vi "PM5000_v3.vi"() -> ()   [LabVIEW 2018]
uses:
  <vilib>/addons/database/Connection.llb/DB Tools Open Connec (Path).vi
  Global/Demo.vi
  Global/estadoGeneradores.vi
  <vilib>/addons/database/NI_Database_API.lvlib
panel:
  out "codeG6":i32
  out "codeG5":i32
  out "codeG4":i32
  out "codeG3":i32
  out "codeG2":i32
  out "codeG1":i32
  out "G6":string
  out "G5":string
  out "G4":string
  out "G3":string
  out "G2":string
  out "G1":string
  out "ID G6":i32
  out "ID G5":i32
  out "ID G4":i32
  out "ID G3":i32
  out "ID G2":i32
  out "ID_G1":i32
  out "error out":errorcluster
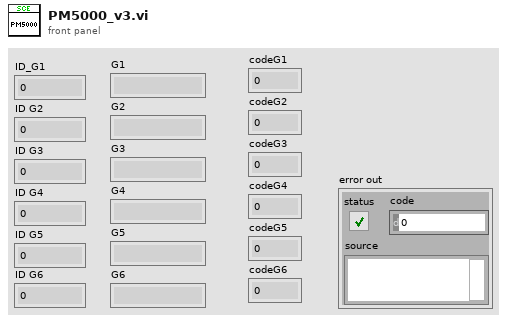
[diagram p1: front panel]
types:
  T1 = typedef "NI_Database_API.lvlib/Conn ObjectReference.ctl" = refnum<k1>
  T2 = typedef "Equipos_Medicion_cluster.ctl" = cluster{"ID_EQUIPO":i32, "IP_EQUIPO":string, "NOMBRE_EQUIPO":string, "ESTADO_EQUIPO":string, "DESCRIPCION":string, "ID_MEDICION":i32, "ESTADO_MEDICION":string, "TIEMPO_MEDICION":string}
  T3 = typedef "Cluster_Data.ctl" = cluster{"Equipo_Medicion":T2, "VIF_cluster":T4, "Power_cluster":T5, "THD_cluster":T6, "Polar_cluster":T7}
  T4 = typedef "VIF_cluster.ctl" = cluster{"VL_VL":cluster{"V1_V2":sgl, "V2_V3":sgl, "V3_V1":sgl, "Avg_VL_VL":sgl}, "IL_IL":cluster{"I1":sgl, "I2":sgl, "I3":sgl, "Avg_Amps":sgl}, "Frecuency":sgl, "Avg_Frecuency":sgl}
  T5 = typedef "Power_cluster.ctl" = cluster{"Real Power (kW)":cluster{"L1_kW":sgl, "L2_kW":sgl, "L3_kW":sgl, "Total_kW":sgl}, "Reactive Power (kVAR)":cluster{"L1_kVAR":sgl, "L2_kVAR":sgl, "L3_kVAR":sgl, "Total_kVAR":sgl}, "Aparent Power (kVA)":cluster{"L1_kVA":sgl, "L2_kVA":sgl, "L3_kVA":sgl, "Total_kVA":sgl}, "Power Factor (%)":cluster{"L1_PF":sgl, "L2_PF":sgl, "L3_PF":sgl, "Total_PF":sgl}}
  T6 = typedef "THD_cluster.ctl" = cluster{"V_THD":cluster{"V1_V2_THD":sgl, "V2_V3_THD":sgl, "V3_V1_THD":sgl, "Avg_V_V_THD":sgl}, "I_THD":cluster{"I1_THD":sgl, "I2_THD":sgl, "I3_THD":sgl, "I4_THD":sgl, "Avg_I_THD":sgl}}
  T7 = typedef "Polar_cluster.ctl" = cluster{"V_polar":cluster{"V1_ang":sgl, "V1_mag":sgl, "V2_ang":sgl, "V2_mag":sgl, "V3_ang":sgl, "V3_mag":sgl}, "I_polar":cluster{"I1_ang":sgl, "I1_mag":sgl, "I2_ang":sgl, "I2_mag":sgl, "I3_ang":sgl, "I3_mag":sgl}}
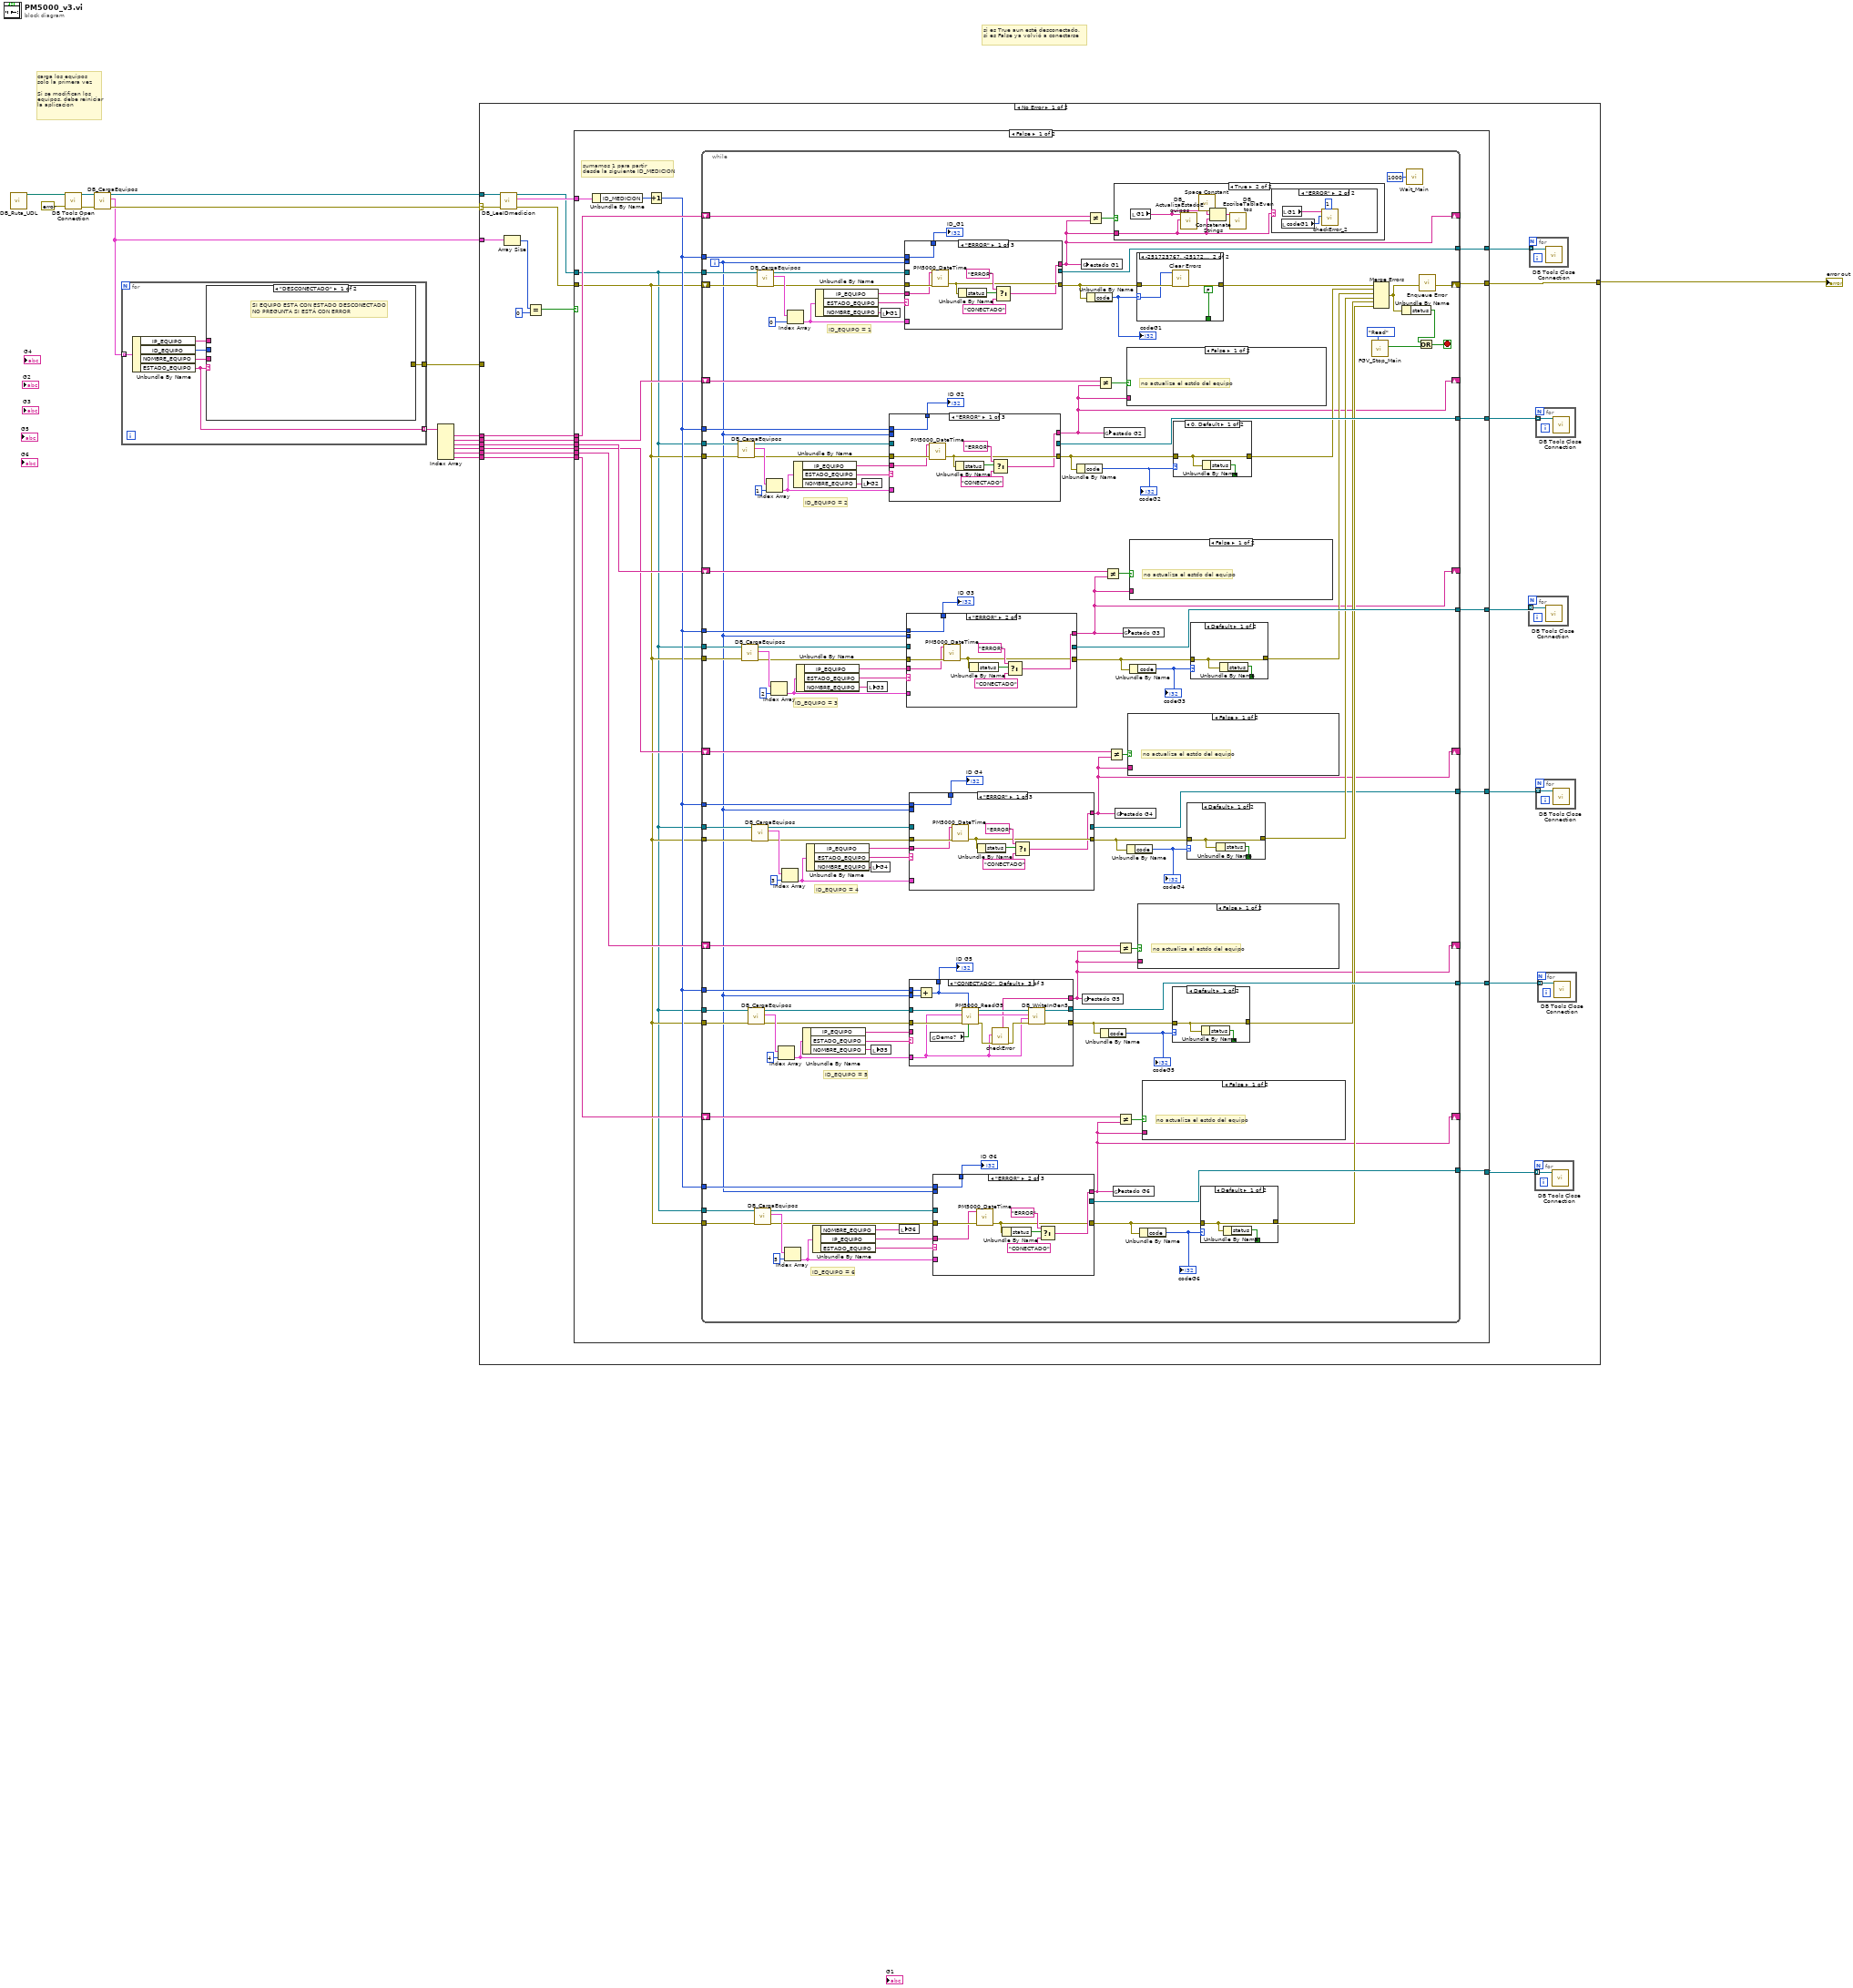
[diagram p0: block diagram]
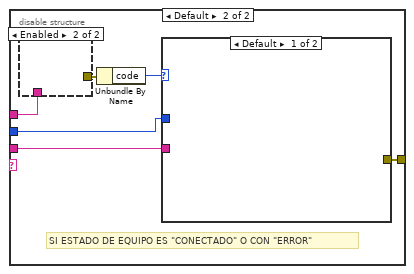
[diagram p2: hidden frame]
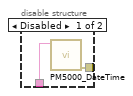
[diagram p3: hidden frame]
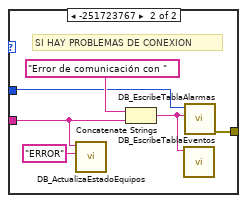
[diagram p4: hidden frame]
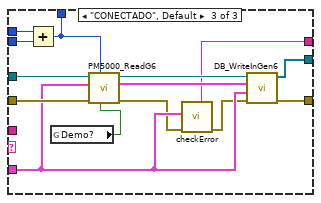
[diagram p6: hidden frame]
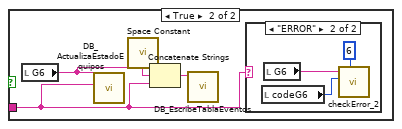
[diagram p7: hidden frame]
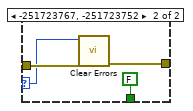
[diagram p9: hidden frame]
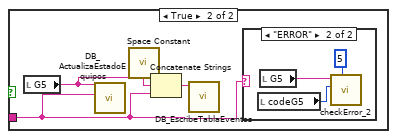
[diagram p10: hidden frame]
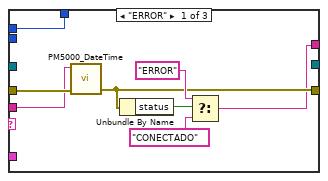
[diagram p12: hidden frame]
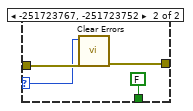
[diagram p14: hidden frame]
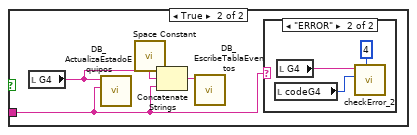
[diagram p15: hidden frame]
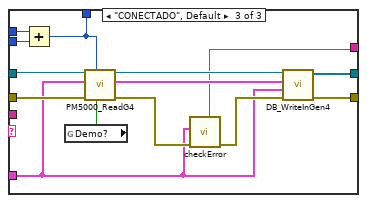
[diagram p18: hidden frame]
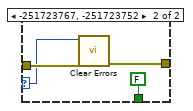
[diagram p19: hidden frame]
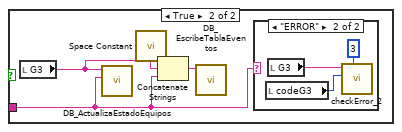
[diagram p20: hidden frame]
diagram:
  # "si es True aun esté desconectado.\nsi es False ya volvió a conectarse"
  # "carga los equipos\nsolo la primera vez\n\nSi se modifican los\nequipos, debe reiniciar\nla aplicacion"
  n1 = call "DB_Ruta_UDL.vi"() -> ("UDL ruta"=w14:path)  [unwired: 11 in]
  n2 = call-poly <vilib>:"DB Tools Open Connection.vi"("error in (no error)"=errorcluster {"status"=FALSE, "code"=0, "source"=""}, "connection information"=w14) -> ("error out"=w12:errorcluster, "connection reference"=w13:T1)  [unwired: 6 in]
  n3 = call "DB_CargaEquipos.vi"("error in (no error)"=w12, "db in"=w13) -> ("error out"=w10:errorcluster, "Equipos_out"=w9:T2[], "db out"=w11:T1)  [unwired: 2 in, 5 out]
  n4 = for {
    tunnel: w9 -> [w22] mode=indexing
    tunnel: [w20] -> w8
    tunnel: [w17] -> w7 mode=indexing
    n5 = Unbundle By Name(w22) -> ("IP_EQUIPO"=w19:string, "ID_EQUIPO"=w21:i32, "NOMBRE_EQUIPO"=w18:string, "ESTADO_EQUIPO"=w17:string)
    n6 = case shown="\"DESCONECTADO\"" w17 {
      tunnel: w21 -> [_ w26]
      tunnel: [_ w25] -> w20
      tunnel: w19 -> [_ w24]
      tunnel: w18 -> [_ w23]
      frame "DESCONECTADO" {
        # "SI EQUIPO ESTA CON ESTADO DESCONECTADO\nNO PREGUNTA SI ESTÁ CON ERROR"
      }
      frame Default {
        # "SI ESTADO DE EQUIPO ES \"CONECTADO\" O CON \"ERROR\""
        n7 = disable-structure shown="Enabled" {
          disable-tunnel: [w30 _] -> w28
          disable-tunnel: w24 -> [w29 _]
          frame Disabled {
            n8 = call "PM5000_DateTime.vi"("Network Path"=w29) -> ("error out"=w30:errorcluster)  [unwired: 7 in, 3 out]
          }
          frame Enabled {
          }
        }
        n9 = Unbundle By Name(w28) -> ("code"=w27:i32)
        n10 = case shown="Default" w27 {
          tunnel: w23 -> [_ w31]
          tunnel: w26 -> [_ w34]
          tunnel: [_ w33] -> w25
          frame Default {
          }
          frame -251723767 {
            # "SI HAY PROBLEMAS DE CONEXION"
            n11 = call "DB_ActualizaEstadoEquipos.vi"("ESTADO_EQUIPO"="ERROR", "NOMBRE_EQUIPO"=w31) -> ()  [unwired: 9 in, 1 out]
            n12 = Concatenate Strings("Error de comunicación con " ("string"), w31) -> (w35:string)
            n13 = call "DB_EscribeTablaEventos.vi"("DESCRIPCION"=w35) -> ()  [unwired: 10 in, 1 out]
            n14 = call "DB_EscribeTablaAlarmas.vi"("MOTIVO"=w35, "ID_EQUIPO"=w34) -> ("error out"=w33:errorcluster)  [unwired: 9 in]
          }
        }
      }
    }
  }
  n15 = Index Array(array=w7) -> (element #1=w5:string, element #2=w4:string, element #3=w3:string, element #4=w2:string, element #5=w1:string, element #6=w6:string)  [unwired: 6 in]
  n16 = case shown="No Error" w10 {
    selector: w10 -> [w44 w428]
    tunnel: [w58 w427] -> w15
    tunnel: w9 -> [w55 _]
    tunnel: w11 -> [w51 _]
    tunnel: w8 -> [_ _]
    tunnel: w6 -> [w43 _]
    tunnel: w5 -> [w41 _]
    tunnel: w4 -> [w40 _]
    tunnel: w3 -> [w39 _]
    tunnel: w2 -> [w38 _]
    tunnel: w1 -> [w37 _]
    frame No Error {
      n17 = call "DB_LeeIDmedicion.vi"("error in (no error)"=w44, "db in"=w51) -> ("error out"=w46:errorcluster, "Equipo_Medicion out"=w50:T2, "db out"=w45:T1)  [unwired: 7 in]
      n18 = Array Size(array=w55) -> (size(s)=w56:i32)
      n19 = Equal?(x=w56, y=0) -> (x = y?=w54:bool)
      n20 = case shown="False" w54 {
        tunnel: [w75 w426] -> w58
        tunnel: w46 -> [w66 w426]
        tunnel: w45 -> [w65 _]
        tunnel: [w82 _] -> w53
        tunnel: [w81 _] -> w52
        tunnel: w50 -> [w80 _]
        tunnel: [w78 _] -> w49
        tunnel: [w77 _] -> w48
        tunnel: [w76 _] -> w47
        tunnel: w43 -> [w74 _]
        tunnel: [w73 _] -> w42
        tunnel: w41 -> [w72 _]
        tunnel: w40 -> [w71 _]
        tunnel: w39 -> [w70 _]
        tunnel: w38 -> [w69 _]
        tunnel: w37 -> [w68 _]
        frame False {
          # "sumamos 1 para partir\ndesde la siguiente ID_MEDICION"
          n21 = Unbundle By Name(w80) -> ("ID_MEDICION"=w79:i32)
          n22 = Increment(x=w79) -> (x+1=w67:i32)
          n23 = while {
            tunnel: [w204] -> w82
            tunnel: [w203] -> w81
            tunnel: [w202] -> w78
            tunnel: [w201] -> w77
            tunnel: [w200] -> w76
            tunnel: w65 -> [w199]
            tunnel: [w189] -> w73
            tunnel: w67 -> [w112]
            shift-right: [w197] -> w75
            shift-left: w66 -> [w198]
            tunnel: w67 -> [w110]
            tunnel: w67 -> [w106]
            tunnel: w67 -> [w105]
            tunnel: w67 -> [w104]
            tunnel: w67 -> [w103]
            tunnel: w66 -> [w102]
            tunnel: w66 -> [w101]
            tunnel: w66 -> [w100]
            tunnel: w66 -> [w99]
            tunnel: w66 -> [w98]
            tunnel: w65 -> [w97]
            tunnel: w65 -> [w96]
            tunnel: w65 -> [w95]
            tunnel: w65 -> [w94]
            tunnel: w65 -> [w93]
            shift-right: [w91] -> _
            shift-left: w72 -> [w188]
            shift-right: [w90] -> _
            shift-left: w71 -> [w187]
            shift-right: [w89] -> _
            shift-left: w70 -> [w186]
            shift-right: [w88] -> _
            shift-left: w69 -> [w185]
            shift-right: [w87] -> _
            shift-left: w68 -> [w184]
            shift-right: [w86] -> _
            shift-left: w74 -> [w190]
            i -> [w92]
            stop <- w107 stop-if-true
            # "ID_EQUIPO = 6"
            # "ID_EQUIPO = 5"
            # "ID_EQUIPO = 4"
            # "ID_EQUIPO = 3"
            # "ID_EQUIPO = 2"
            # "ID_EQUIPO = 1"
            n24 = call "DB_CargaEquipos.vi"("error in (no error)"=w102, "db in"=w97) -> ("error out"=w168:errorcluster, "Equipos_out"=w171:T2[], "db out"=w170:T1)  [unwired: 2 in, 5 out]
            n25 = call "DB_CargaEquipos.vi"("error in (no error)"=w101, "db in"=w96) -> ("error out"=w156:errorcluster, "Equipos_out"=w159:T2[], "db out"=w158:T1)  [unwired: 2 in, 5 out]
            n26 = call "DB_CargaEquipos.vi"("error in (no error)"=w99, "db in"=w94) -> ("error out"=w134:errorcluster, "Equipos_out"=w137:T2[], "db out"=w136:T1)  [unwired: 2 in, 5 out]
            n27 = call "DB_CargaEquipos.vi"("error in (no error)"=w100, "db in"=w95) -> ("error out"=w145:errorcluster, "Equipos_out"=w148:T2[], "db out"=w147:T1)  [unwired: 2 in, 5 out]
            n28 = call "DB_CargaEquipos.vi"("error in (no error)"=w98, "db in"=w93) -> ("error out"=w120:errorcluster, "Equipos_out"=w123:T2[], "db out"=w122:T1)  [unwired: 2 in, 5 out]
            n29 = call "DB_CargaEquipos.vi"("error in (no error)"=w198, "db in"=w199) -> ("error out"=w179:errorcluster, "Equipos_out"=w182:T2[], "db out"=w181:T1)  [unwired: 2 in, 5 out]
            n30 = Index Array(array=w171, index=1) -> (element=w167:T2)
            n31 = Index Array(array=w159, index=2) -> (element=w155:T2)
            n32 = Index Array(array=w137, index=4) -> (element=w133:T2)
            n33 = Index Array(array=w148, index=3) -> (element=w144:T2)
            n34 = Index Array(array=w123, index=5) -> (element=w119:T2)
            n35 = Index Array(array=w182, index=0) -> (element=w178:T2)
            n36 = Unbundle By Name(w167) -> ("IP_EQUIPO"=w164:string, "ESTADO_EQUIPO"=w166:string, "NOMBRE_EQUIPO"=w161:string)
            n37 = Unbundle By Name(w155) -> ("IP_EQUIPO"=w152:string, "ESTADO_EQUIPO"=w154:string, "NOMBRE_EQUIPO"=w150:string)
            n38 = Unbundle By Name(w133) -> ("IP_EQUIPO"=w130:string, "ESTADO_EQUIPO"=w132:string, "NOMBRE_EQUIPO"=w126:string)
            n39 = Unbundle By Name(w144) -> ("IP_EQUIPO"=w142:string, "ESTADO_EQUIPO"=w143:string, "NOMBRE_EQUIPO"=w140:string)
            n40 = Unbundle By Name(w119) -> ("NOMBRE_EQUIPO"=w116:string, "IP_EQUIPO"=w117:string, "ESTADO_EQUIPO"=w118:string)
            n41 = Unbundle By Name(w178) -> ("IP_EQUIPO"=w176:string, "ESTADO_EQUIPO"=w177:string, "NOMBRE_EQUIPO"=w175:string)
            n42 = local write "G2"(w161) -> ()
            n43 = local write "G3"(w150) -> ()
            n44 = local write "G4"(w140) -> ()
            n45 = local write "G5"(w126) -> ()
            n46 = local write "G1"(w175) -> ()
            n47 = case shown="\"ERROR\"" w166 {
              selector: w166 -> [_ w369 _]
              tunnel: [_ _ w382] -> w203
              tunnel: w170 -> [_ _ w380]
              tunnel: w167 -> [_ _ w373]
              tunnel: [w367 w368 w376] -> w165
              tunnel: w168 -> [w363 _ w379]
              tunnel: [w361 _ w378] -> w172
              tunnel: [w360 w369 w372] -> w90
              tunnel: w112 -> [w367 w368 w377]
              tunnel: w164 -> [w362 _ _]
              tunnel: w92 -> [_ _ w371]
              frame "ERROR" {
                n48 = call "PM5000_DateTime.vi"("error in"=w363, "Network Path"=w362) -> ("error out"=w361:errorcluster)  [unwired: 6 in, 3 out]
                n49 = Unbundle By Name(w361) -> ("status"=w366:bool)
                n50 = Select(t="ERROR", s=w366, f="CONECTADO") -> (s? t:f=w360:string)
              }
              frame "DESCONECTADO" {
              }
              frame "CONECTADO", Default {
                n51 = Add(x=w377, y=w371) -> (x+y=w376:i32)
                n52 = global read "Demo.vi" "Demo?"() -> (w370:bool)
                n53 = call "PM5000_ReadG2.vi"("DEMO"=w370, "ID_MEDICION"=w376, "error in (no error)"=w379, "Equipo_Medicion"=w373) -> ("error out"=w375:errorcluster, "PM_out"=w381:T3)  [unwired: 6 in]
                n54 = call "checkError.vi"("error in (no error)"=w375, "Equipo_Medicion in"=w373) -> ("error out"=w374:errorcluster, "ESTADO_EQUIPO"=w372:string)  [unwired: 8 in]
                n55 = call "DB_WriteInGen2.vi"("error in (no error)"=w374, "Equipo_Medicion"=w373, "PM_out"=w381, "DB in"=w380) -> ("error out"=w378:errorcluster, "closeDB"=w382:T1[])  [unwired: 6 in]
              }
            }
            "ID G2" <- w165
            n56 = local write "G6"(w116) -> ()
            n57 = case shown="\"ERROR\"" w177 {
              selector: w177 -> [_ w406 _]
              tunnel: [_ _ w419] -> w204
              tunnel: w181 -> [_ _ w418]
              tunnel: w179 -> [w400 w405 w416]
              tunnel: [w399 w405 w415] -> w183
              tunnel: w178 -> [_ _ w408]
              tunnel: w176 -> [w396 _ _]
              tunnel: [w398 w406 w412] -> w91
              tunnel: [w397 w404 w411] -> w113
              tunnel: w110 -> [w397 w404 w410]
              tunnel: w92 -> [_ _ w409]
              frame "ERROR" {
                n58 = call "PM5000_DateTime.vi"("error in"=w400, "Network Path"=w396) -> ("error out"=w399:errorcluster)  [unwired: 6 in, 3 out]
                n59 = Unbundle By Name(w399) -> ("status"=w403:bool)
                n60 = Select(t="ERROR", s=w403, f="CONECTADO") -> (s? t:f=w398:string)
              }
              frame "DESCONECTADO" {
              }
              frame "CONECTADO", Default {
                n61 = Add(x=w410, y=w409) -> (x+y=w411:i32)
                n62 = global read "Demo.vi" "Demo?"() -> (w407:bool)
                n63 = call "PM5000_ReadG1.vi"("DEMO"=w407, "ID_MEDICION"=w411, "error in (no error)"=w416, "Equipo_Medicion"=w408) -> ("error out"=w414:errorcluster, "PM_out"=w417:T3)  [unwired: 6 in]
                n64 = call "checkError.vi"("error in (no error)"=w414, "Equipo_Medicion in"=w408) -> ("error out"=w413:errorcluster, "ESTADO_EQUIPO"=w412:string)  [unwired: 8 in]
                n65 = call "DB_WriteInGen1.vi"("error in (no error)"=w413, "Equipo_Medicion"=w408, "PM_out"=w417, "DB in"=w418) -> ("error out"=w415:errorcluster, "closeDB"=w419:T1[])  [unwired: 6 in]
              }
            }
            "ID_G1" <- w113
            n66 = case shown="\"ERROR\"" w154 {
              selector: w154 -> [_ _ w346]
              tunnel: [w335 _ _] -> w202
              tunnel: w158 -> [w333 _ _]
              tunnel: w155 -> [w326 _ _]
              tunnel: w156 -> [w332 w340 w345]
              tunnel: [w331 w337 w345] -> w160
              tunnel: [w327 w338 w346] -> w89
              tunnel: [w330 w336 w344] -> w153
              tunnel: w152 -> [_ w339 _]
              tunnel: w106 -> [w325 w336 w344]
              tunnel: w92 -> [w324 _ _]
              frame "CONECTADO", Default {
                n67 = Add(x=w325, y=w324) -> (x+y=w330:i32)
                n68 = global read "Demo.vi" "Demo?"() -> (w323:bool)
                n69 = call "PM5000_ReadG3.vi"("DEMO"=w323, "ID_MEDICION"=w330, "error in (no error)"=w332, "Equipo_Medicion"=w326) -> ("error out"=w329:errorcluster, "PM_out"=w334:T3)  [unwired: 6 in]
                n70 = call "checkError.vi"("error in (no error)"=w329, "Equipo_Medicion in"=w326) -> ("error out"=w328:errorcluster, "ESTADO_EQUIPO"=w327:string)  [unwired: 8 in]
                n71 = call "DB_WriteInGen3.vi"("error in (no error)"=w328, "Equipo_Medicion"=w326, "PM_out"=w334, "DB in"=w333) -> ("error out"=w331:errorcluster, "closeDB"=w335:T1[])  [unwired: 6 in]
              }
              frame "ERROR" {
                n72 = call "PM5000_DateTime.vi"("error in"=w340, "Network Path"=w339) -> ("error out"=w337:errorcluster)  [unwired: 6 in, 3 out]
                n73 = Unbundle By Name(w337) -> ("status"=w343:bool)
                n74 = Select(t="ERROR", s=w343, f="CONECTADO") -> (s? t:f=w338:string)
              }
              frame "DESCONECTADO" {
              }
            }
            "ID G3" <- w153
            n75 = case shown="\"CONECTADO\", Default" w132 {
              selector: w132 -> [_ w258 _]
              tunnel: [_ _ w272] -> w201
              tunnel: w136 -> [_ _ w270]
              tunnel: w133 -> [_ _ w264]
              tunnel: w134 -> [w253 w259 w269]
              tunnel: [w251 w259 w268] -> w129
              tunnel: [w250 w258 w263] -> w87
              tunnel: [w249 w257 w267] -> w131
              tunnel: w130 -> [w252 _ _]
              tunnel: w104 -> [w249 w257 w262]
              tunnel: w92 -> [_ _ w261]
              frame "ERROR" {
                n76 = call "PM5000_DateTime.vi"("error in"=w253, "Network Path"=w252) -> ("error out"=w251:errorcluster)  [unwired: 6 in, 3 out]
                n77 = Unbundle By Name(w251) -> ("status"=w256:bool)
                n78 = Select(t="ERROR", s=w256, f="CONECTADO") -> (s? t:f=w250:string)
              }
              frame "DESCONECTADO" {
              }
              frame "CONECTADO", Default {
                n79 = Add(x=w262, y=w261) -> (x+y=w267:i32)
                n80 = global read "Demo.vi" "Demo?"() -> (w260:bool)
                n81 = call "PM5000_ReadG5.vi"("DEMO"=w260, "ID_MEDICION"=w267, "error in (no error)"=w269, "Equipo_Medicion"=w264) -> ("error out"=w266:errorcluster, "PM_out"=w271:T3)  [unwired: 6 in]
                n82 = call "checkError.vi"("error in (no error)"=w266, "Equipo_Medicion in"=w264) -> ("error out"=w265:errorcluster, "ESTADO_EQUIPO"=w263:string)  [unwired: 8 in]
                n83 = call "DB_WriteInGen5.vi"("error in (no error)"=w265, "Equipo_Medicion"=w264, "PM_out"=w271, "DB in"=w270) -> ("error out"=w268:errorcluster, "closeDB"=w272:T1[])  [unwired: 6 in]
              }
            }
            "ID G5" <- w131
            n84 = case shown="\"ERROR\"" w143 {
              selector: w143 -> [_ w296 _]
              tunnel: [_ _ w309] -> w189
              tunnel: w147 -> [_ _ w307]
              tunnel: w144 -> [_ _ w302]
              tunnel: w145 -> [w290 w295 w306]
              tunnel: [w289 w295 w305] -> w139
              tunnel: [w288 w296 w301] -> w88
              tunnel: w142 -> [w287 _ _]
              tunnel: [w286 w294 w300] -> w111
              tunnel: w105 -> [w286 w294 w299]
              tunnel: w92 -> [_ _ w298]
              frame "ERROR" {
                n85 = call "PM5000_DateTime.vi"("error in"=w290, "Network Path"=w287) -> ("error out"=w289:errorcluster)  [unwired: 6 in, 3 out]
                n86 = Unbundle By Name(w289) -> ("status"=w293:bool)
                n87 = Select(t="ERROR", s=w293, f="CONECTADO") -> (s? t:f=w288:string)
              }
              frame "DESCONECTADO" {
              }
              frame "CONECTADO", Default {
                n88 = Add(x=w299, y=w298) -> (x+y=w300:i32)
                n89 = global read "Demo.vi" "Demo?"() -> (w297:bool)
                n90 = call "PM5000_ReadG4.vi"("DEMO"=w297, "ID_MEDICION"=w300, "error in (no error)"=w306, "Equipo_Medicion"=w302) -> ("error out"=w304:errorcluster, "PM_out"=w308:T3)  [unwired: 6 in]
                n91 = call "checkError.vi"("error in (no error)"=w304, "Equipo_Medicion in"=w302) -> ("error out"=w303:errorcluster, "ESTADO_EQUIPO"=w301:string)  [unwired: 8 in]
                n92 = call "DB_WriteInGen4.vi"("error in (no error)"=w303, "Equipo_Medicion"=w302, "PM_out"=w308, "DB in"=w307) -> ("error out"=w305:errorcluster, "closeDB"=w309:T1[])  [unwired: 6 in]
              }
            }
            "ID G4" <- w111
            n93 = case shown="\"ERROR\"" w118 {
              selector: w118 -> [w207 _ _]
              tunnel: [_ _ w228] -> w200
              tunnel: w122 -> [_ _ w226]
              tunnel: w119 -> [_ _ w224]
              tunnel: w120 -> [w206 w215 w225]
              tunnel: [w206 w209 w220] -> w125
              tunnel: [w207 w210 w223] -> w86
              tunnel: w117 -> [_ w214 _]
              tunnel: [w205 w208 w219] -> w114
              tunnel: w103 -> [w205 w208 w218]
              tunnel: w92 -> [_ _ w217]
              frame "DESCONECTADO" {
              }
              frame "ERROR" {
                n94 = call "PM5000_DateTime.vi"("error in"=w215, "Network Path"=w214) -> ("error out"=w209:errorcluster)  [unwired: 6 in, 3 out]
                n95 = Unbundle By Name(w209) -> ("status"=w213:bool)
                n96 = Select(t="ERROR", s=w213, f="CONECTADO") -> (s? t:f=w210:string)
              }
              frame "CONECTADO", Default {
                n97 = Add(x=w218, y=w217) -> (x+y=w219:i32)
                n98 = global read "Demo.vi" "Demo?"() -> (w216:bool)
                n99 = call "PM5000_ReadG6.vi"("DEMO"=w216, "ID_MEDICION"=w219, "error in (no error)"=w225, "Equipo_Medicion"=w224) -> ("error out"=w222:errorcluster, "PM_out"=w227:T3)  [unwired: 6 in]
                n100 = call "checkError.vi"("error in (no error)"=w222, "Equipo_Medicion in"=w224) -> ("error out"=w221:errorcluster, "ESTADO_EQUIPO"=w223:string)  [unwired: 8 in]
                n101 = call "DB_WriteInGen6.vi"("error in (no error)"=w221, "Equipo_Medicion"=w224, "PM_out"=w227, "DB in"=w226) -> ("error out"=w220:errorcluster, "closeDB"=w228:T1[])  [unwired: 6 in]
              }
            }
            "ID G6" <- w114
            n102 = Unbundle By Name(w172) -> ("code"=w163:i32)
            "codeG2" <- w163
            n103 = global write "estadoGeneradores.vi" "estado G1"(w91) -> ()
            n104 = global write "estadoGeneradores.vi" "estado G5"(w87) -> ()
            n105 = Unbundle By Name(w183) -> ("code"=w174:i32)
            "codeG1" <- w174
            n106 = Not Equal?(x=w188, y=w91) -> (x != y?=w173:bool)
            n107 = Not Equal?(x=w187, y=w90) -> (x != y?=w162:bool)
            n108 = Unbundle By Name(w129) -> ("code"=w128:i32)
            "codeG5" <- w128
            n109 = global write "estadoGeneradores.vi" "estado G2"(w90) -> ()
            n110 = Not Equal?(x=w186, y=w89) -> (x != y?=w149:bool)
            n111 = Not Equal?(x=w185, y=w88) -> (x != y?=w141:bool)
            n112 = global write "estadoGeneradores.vi" "estado G6"(w86) -> ()
            n113 = case shown="True" w173 {
              tunnel: w91 -> [_ w389]
              frame False {
                # "no actualiza el estdo del equipo"
              }
              frame True {
                n114 = local read "G1"() -> (w390:string)
                n115 = call "DB_ActualizaEstadoEquipos.vi"("ESTADO_EQUIPO"=w389, "NOMBRE_EQUIPO"=w390) -> ()  [unwired: 9 in, 1 out]
                n116 = call <vilib>:"Space Constant.vi"() -> ("String"=w391:string)
                n117 = Concatenate Strings(w390, w391, w389) -> (w392:string)
                n118 = call "DB_EscribeTablaEventos.vi"("DESCRIPCION"=w392) -> ()  [unwired: 10 in, 1 out]
                n119 = case shown="\"ERROR\"" w389 {
                  frame Default {
                  }
                  frame "ERROR" {
                    n120 = local read "codeG1"() -> (w394:i32)
                    n121 = local read "G1"() -> (w395:string)
                    n122 = call "checkError_2.vi"("ID_EQUIPO"=1, "code_IN"=w394, "Gen_IN"=w395) -> ()  [unwired: 9 in]
                  }
                }
              }
            }
            n123 = global write "estadoGeneradores.vi" "estado G4"(w88) -> ()
            n124 = Not Equal?(x=w184, y=w87) -> (x != y?=w127:bool)
            n125 = Not Equal?(x=w190, y=w86) -> (x != y?=w124:bool)
            n126 = global write "estadoGeneradores.vi" "estado G3"(w89) -> ()
            n127 = case shown="False" w162 {
              tunnel: w90 -> [_ w353]
              frame False {
                # "no actualiza el estdo del equipo"
              }
              frame True {
                n128 = local read "G2"() -> (w354:string)
                n129 = call "DB_ActualizaEstadoEquipos.vi"("ESTADO_EQUIPO"=w353, "NOMBRE_EQUIPO"=w354) -> ()  [unwired: 9 in, 1 out]
                n130 = call <vilib>:"Space Constant.vi"() -> ("String"=w355:string)
                n131 = Concatenate Strings(w354, w355, w353) -> (w356:string)
                n132 = call "DB_EscribeTablaEventos.vi"("DESCRIPCION"=w356) -> ()  [unwired: 10 in, 1 out]
                n133 = case shown="\"ERROR\"" w353 {
                  frame Default {
                  }
                  frame "ERROR" {
                    n134 = local read "codeG2"() -> (w358:i32)
                    n135 = local read "G2"() -> (w359:string)
                    n136 = call "checkError_2.vi"("ID_EQUIPO"=2, "code_IN"=w358, "Gen_IN"=w359) -> ()  [unwired: 9 in]
                  }
                }
              }
            }
            n137 = Unbundle By Name(w139) -> ("code"=w138:i32)
            "codeG4" <- w138
            n138 = case shown="False" w141 {
              tunnel: w88 -> [_ w279]
              frame False {
                # "no actualiza el estdo del equipo"
              }
              frame True {
                n139 = local read "G4"() -> (w280:string)
                n140 = call "DB_ActualizaEstadoEquipos.vi"("ESTADO_EQUIPO"=w279, "NOMBRE_EQUIPO"=w280) -> ()  [unwired: 9 in, 1 out]
                n141 = call <vilib>:"Space Constant.vi"() -> ("String"=w281:string)
                n142 = Concatenate Strings(w280, w281, w279) -> (w282:string)
                n143 = call "DB_EscribeTablaEventos.vi"("DESCRIPCION"=w282) -> ()  [unwired: 10 in, 1 out]
                n144 = case shown="\"ERROR\"" w279 {
                  frame Default {
                  }
                  frame "ERROR" {
                    n145 = local read "codeG4"() -> (w284:i32)
                    n146 = local read "G4"() -> (w285:string)
                    n147 = call "checkError_2.vi"("ID_EQUIPO"=4, "code_IN"=w284, "Gen_IN"=w285) -> ()  [unwired: 9 in]
                  }
                }
              }
            }
            n148 = case shown="False" w149 {
              tunnel: w89 -> [_ w316]
              frame False {
                # "no actualiza el estdo del equipo"
              }
              frame True {
                n149 = local read "G3"() -> (w317:string)
                n150 = call "DB_ActualizaEstadoEquipos.vi"("ESTADO_EQUIPO"=w316, "NOMBRE_EQUIPO"=w317) -> ()  [unwired: 9 in, 1 out]
                n151 = call <vilib>:"Space Constant.vi"() -> ("String"=w318:string)
                n152 = Concatenate Strings(w317, w318, w316) -> (w319:string)
                n153 = call "DB_EscribeTablaEventos.vi"("DESCRIPCION"=w319) -> ()  [unwired: 10 in, 1 out]
                n154 = case shown="\"ERROR\"" w316 {
                  frame Default {
                  }
                  frame "ERROR" {
                    n155 = local read "codeG3"() -> (w321:i32)
                    n156 = local read "G3"() -> (w322:string)
                    n157 = call "checkError_2.vi"("ID_EQUIPO"=3, "code_IN"=w321, "Gen_IN"=w322) -> ()  [unwired: 9 in]
                  }
                }
              }
            }
            n158 = Unbundle By Name(w160) -> ("code"=w151:i32)
            "codeG3" <- w151
            n159 = case shown="-251723767, -251723752" w174 {
              selector: w174 -> [_ w422]
              tunnel: [w421 w425] -> w196
              tunnel: w183 -> [w421 w424]
              tunnel: [w420 FALSE ("status")] -> _
              frame Default {
                n160 = Unbundle By Name(w421) -> ("status"=w420:bool)
              }
              frame -251723767, -251723752 {
                n161 = call <vilib>:"Clear Errors.vi"("error in (no error)"=w424, "specific error code to clear (0: all)"=w422) -> ("error out"=w425:errorcluster)  [unwired: 4 in, 1 out]
              }
            }
            n162 = case shown="False" w127 {
              tunnel: w87 -> [_ w242]
              frame False {
                # "no actualiza el estdo del equipo"
              }
              frame True {
                n163 = local read "G5"() -> (w243:string)
                n164 = call "DB_ActualizaEstadoEquipos.vi"("ESTADO_EQUIPO"=w242, "NOMBRE_EQUIPO"=w243) -> ()  [unwired: 9 in, 1 out]
                n165 = call <vilib>:"Space Constant.vi"() -> ("String"=w244:string)
                n166 = Concatenate Strings(w243, w244, w242) -> (w245:string)
                n167 = call "DB_EscribeTablaEventos.vi"("DESCRIPCION"=w245) -> ()  [unwired: 10 in, 1 out]
                n168 = case shown="\"ERROR\"" w242 {
                  frame Default {
                  }
                  frame "ERROR" {
                    n169 = local read "codeG5"() -> (w248:i32)
                    n170 = local read "G5"() -> (w247:string)
                    n171 = call "checkError_2.vi"("ID_EQUIPO"=5, "code_IN"=w248, "Gen_IN"=w247) -> ()  [unwired: 9 in]
                  }
                }
              }
            }
            n172 = Unbundle By Name(w125) -> ("code"=w115:i32)
            "codeG6" <- w115
            n173 = case shown="False" w124 {
              tunnel: w86 -> [_ w229]
              frame False {
                # "no actualiza el estdo del equipo"
              }
              frame True {
                n174 = local read "G6"() -> (w230:string)
                n175 = call "DB_ActualizaEstadoEquipos.vi"("ESTADO_EQUIPO"=w229, "NOMBRE_EQUIPO"=w230) -> ()  [unwired: 9 in, 1 out]
                n176 = call <vilib>:"Space Constant.vi"() -> ("String"=w231:string)
                n177 = Concatenate Strings(w230, w231, w229) -> (w232:string)
                n178 = call "DB_EscribeTablaEventos.vi"("DESCRIPCION"=w232) -> ()  [unwired: 10 in, 1 out]
                n179 = case shown="\"ERROR\"" w229 {
                  frame Default {
                  }
                  frame "ERROR" {
                    n180 = local read "codeG6"() -> (w235:i32)
                    n181 = local read "G6"() -> (w234:string)
                    n182 = call "checkError_2.vi"("ID_EQUIPO"=6, "code_IN"=w235, "Gen_IN"=w234) -> ()  [unwired: 9 in]
                  }
                }
              }
            }
            n183 = case shown="Default" w128 {
              selector: w128 -> [_ w275]
              tunnel: [w273 FALSE ("status")] -> _
              tunnel: [w274 w278] -> w193
              tunnel: w129 -> [w274 w276]
              frame Default {
                n184 = Unbundle By Name(w274) -> ("status"=w273:bool)
              }
              frame -251723767, -251723752 {
                n185 = call <vilib>:"Clear Errors.vi"("error in (no error)"=w276, "specific error code to clear (0: all)"=w275) -> ("error out"=w278:errorcluster)  [unwired: 4 in, 1 out]
              }
            }
            n186 = case shown="0, Default" w163 {
              selector: w163 -> [_ w385]
              tunnel: [w384 FALSE ("status")] -> _
              tunnel: w172 -> [w383 w388]
              tunnel: [w383 w387] -> w195
              frame 0, Default {
                n187 = Unbundle By Name(w383) -> ("status"=w384:bool)
              }
              frame -251723767, -251723752 {
                n188 = call <vilib>:"Clear Errors.vi"("error in (no error)"=w388, "specific error code to clear (0: all)"=w385) -> ("error out"=w387:errorcluster)  [unwired: 4 in, 1 out]
              }
            }
            n189 = case shown="Default" w138 {
              selector: w138 -> [_ w312]
              tunnel: [w310 FALSE ("status")] -> _
              tunnel: [w311 w315] -> w194
              tunnel: w139 -> [w311 w313]
              frame Default {
                n190 = Unbundle By Name(w311) -> ("status"=w310:bool)
              }
              frame -251723767, -251723752 {
                n191 = call <vilib>:"Clear Errors.vi"("error in (no error)"=w313, "specific error code to clear (0: all)"=w312) -> ("error out"=w315:errorcluster)  [unwired: 4 in, 1 out]
              }
            }
            n192 = case shown="Default" w151 {
              selector: w151 -> [_ w349]
              tunnel: [w347 FALSE ("status")] -> _
              tunnel: [w348 w352] -> w191
              tunnel: w160 -> [w348 w350]
              frame Default {
                n193 = Unbundle By Name(w348) -> ("status"=w347:bool)
              }
              frame -251723767, -251723752 {
                n194 = call <vilib>:"Clear Errors.vi"("error in (no error)"=w350, "specific error code to clear (0: all)"=w349) -> ("error out"=w352:errorcluster)  [unwired: 4 in, 1 out]
              }
            }
            n195 = case shown="Default" w115 {
              selector: w115 -> [_ w238]
              tunnel: [w236 FALSE ("status")] -> _
              tunnel: [w237 w241] -> w192
              tunnel: w125 -> [w237 w239]
              frame Default {
                n196 = Unbundle By Name(w237) -> ("status"=w236:bool)
              }
              frame -251723767, -251723752 {
                n197 = call <vilib>:"Clear Errors.vi"("error in (no error)"=w239, "specific error code to clear (0: all)"=w238) -> ("error out"=w241:errorcluster)  [unwired: 4 in, 1 out]
              }
            }
            n198 = call "FGV_Stop_Main.vi"("Action"=enum16{"Read", "Write"}."Read") -> ("Var Out"=w109:bool)  [unwired: 9 in, 1 out]
            n199 = Merge Errors(w196, w195, w191, w194, w193, w192) -> (w85:errorcluster)
            n200 = Unbundle By Name(w85) -> ("status"=w84:bool)
            n201 = call "Wait_Main.vi"("Wait time (msec)"=u32 1000) -> ()  [unwired: 5 in]
            n202 = Or(x=w84, y=w109) -> (x .or. y?=w107:bool)
            n203 = call "Enqueue Error.vi"("error in"=w85) -> ("error out"=w197:errorcluster)  [unwired: 9 in, 1 out]
          }
        }
        frame True {
          # "detiene \nel VI"
          n204 = call "Display Message to User"() -> ()  [unwired: 10 in, 2 out]
        }
      }
      n205 = for {
        tunnel: w49 -> [w62] mode=indexing
        n206 = call <vilib>:"DB Tools Close Connection.vi"("connection reference"=w62) -> ()  [unwired: 6 in, 1 out]
      }
      n207 = for {
        tunnel: w53 -> [w64] mode=indexing
        n208 = call <vilib>:"DB Tools Close Connection.vi"("connection reference"=w64) -> ()  [unwired: 6 in, 1 out]
      }
      n209 = for {
        tunnel: w47 -> [w59] mode=indexing
        n210 = call <vilib>:"DB Tools Close Connection.vi"("connection reference"=w59) -> ()  [unwired: 6 in, 1 out]
      }
      n211 = for {
        tunnel: w52 -> [w63] mode=indexing
        n212 = call <vilib>:"DB Tools Close Connection.vi"("connection reference"=w63) -> ()  [unwired: 6 in, 1 out]
      }
      n213 = for {
        tunnel: w42 -> [w61] mode=indexing
        n214 = call <vilib>:"DB Tools Close Connection.vi"("connection reference"=w61) -> ()  [unwired: 6 in, 1 out]
      }
      n215 = for {
        tunnel: w48 -> [w60] mode=indexing
        n216 = call <vilib>:"DB Tools Close Connection.vi"("connection reference"=w60) -> ()  [unwired: 6 in, 1 out]
      }
    }
    frame Error {
      n217 = call "Enqueue Error.vi"("error in"=w428) -> ("error out"=w427:errorcluster)  [unwired: 9 in, 1 out]
    }
  }
  "error out" <- w15
